vi "IntegerDatetimeToSQLDateTime.vi"(9 "Time":i32, 10 "Date":i32) -> (2 "SQL Datime":string)   [LabVIEW 2012]
uses:
  <vilib>/Utility/miscctls.llb/LVDateTimeRec.ctl
panel:
  in  "date time rec":T1
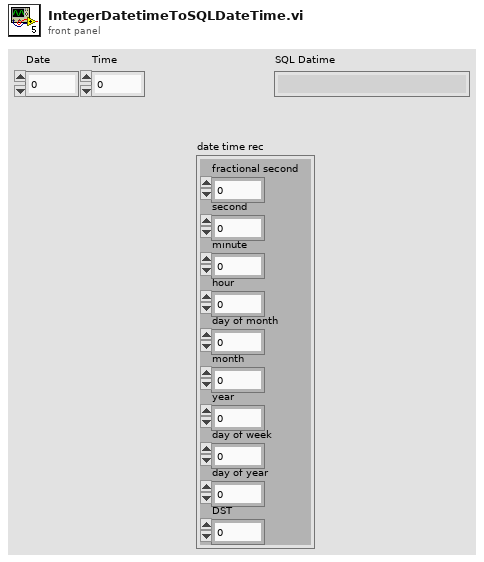
[diagram p1: front panel]
types:
  T1 = typedef "LVDateTimeRec.ctl" = cluster{"fractional second":dbl, "second":i32, "minute":i32, "hour":i32, "day of month":i32, "month":i32, "year":i32, "day of week":i32, "day of year":i32, "DST":i32}
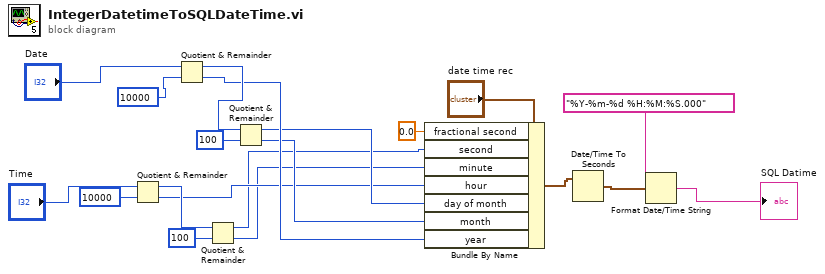
[diagram p0: block diagram]
diagram:
  n1 = Quotient & Remainder(x="Time", y=10000) -> (x-y*floor(x/y)=w8:i32, floor(x/y)=w7:i32)
  n2 = Quotient & Remainder(x="Date", y=10000) -> (x-y*floor(x/y)=w12:i32, floor(x/y)=w11:i32)
  n3 = Quotient & Remainder(x=w8, y=100) -> (x-y*floor(x/y)=w5:i32, floor(x/y)=w6:i32)
  n4 = Quotient & Remainder(x=w12, y=100) -> (x-y*floor(x/y)=w9:i32, floor(x/y)=w10:i32)
  n5 = Bundle By Name(cluster="date time rec", "fractional second"=0.0, "second"=w5, "minute"=w6, "hour"=w7, "day of month"=w9, "month"=w10, "year"=w11) -> (w4:T1)
  n6 = Date/Time To Seconds(2:w4) -> (0:w3:timestamp)  [unwired: 1 in]
  n7 = Format Date/Time String(time format string (%c)="%Y-%m-%d %H:%M:%S.000", seconds (now)=w3) -> (date/time string=→"SQL Datime":string)  [unwired: 1 in]
